vi "DT_GetDependencyFiles.vi"(7 "Framwork Type":T1) -> (1 "rel. Filepaths .js":path[](array[path]), 2 "rel. Filepaths .css":path[](array[path]))   [LabVIEW 2014]
uses:
  controls/StylingFrameworks_Enum.ctl
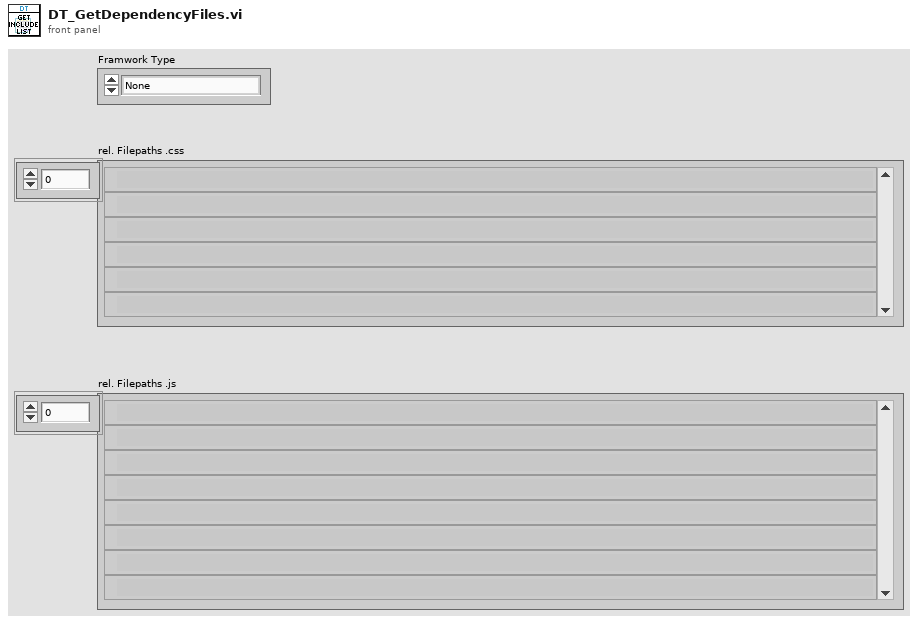
[diagram p1: front panel]
types:
  T1 = typedef "StylingFrameworks_Enum.ctl" = enum16{"None", "Bootstrap4", "Semantic-UI", "Custom"}
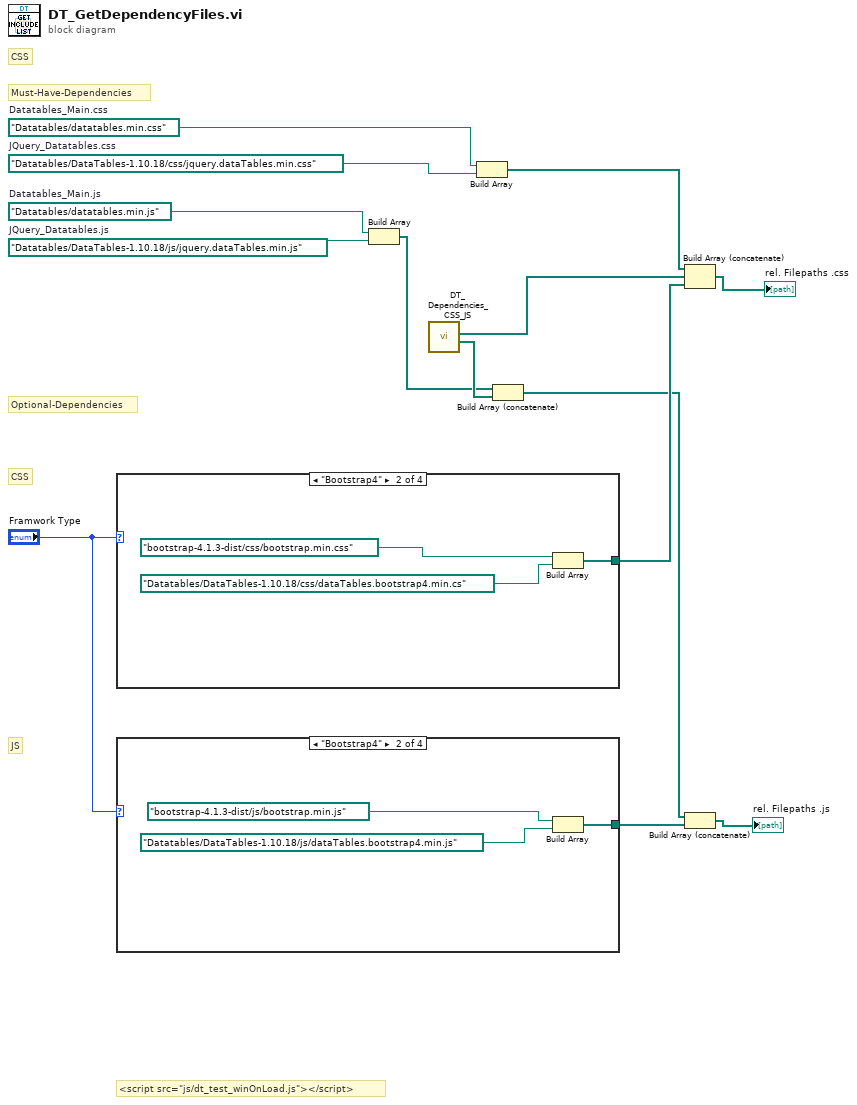
[diagram p0: block diagram]
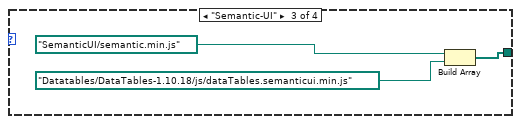
[diagram p3: hidden frame]
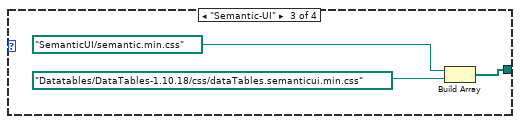
[diagram p6: hidden frame]
diagram:
  w6 = path "Datatables/DataTables-1.10.18/js/jquery.dataTables.min.js"  # JQuery_Datatables.js
  w7 = path "Datatables/datatables.min.js"  # Datatables_Main.js
  w10 = path "Datatables/DataTables-1.10.18/css/jquery.dataTables.min.css"  # JQuery_Datatables.css
  w12 = path "Datatables/datatables.min.css"  # Datatables_Main.css
  # "CSS"
  # "JS"
  # "CSS"
  # "<script src=\"js/dt_test_winOnLoad.js\"></script>"
  # "Optional-Dependencies"
  # "Must-Have-Dependencies"
  n1 = case shown="\"Bootstrap4\"" "Framwork Type" {
    tunnel: [_ w15 w18 _] -> w9
    frame "None", Default {
    }
    frame "Bootstrap4" {
      n2 = Build Array(path "bootstrap-4.1.3-dist/css/bootstrap.min.css", path "Datatables/DataTables-1.10.18/css/dataTables.bootstrap4.min.cs") -> (w15:path[])
    }
    frame "Semantic-UI" {
      n3 = Build Array(path "SemanticUI/semantic.min.css", path "Datatables/DataTables-1.10.18/css/dataTables.semanticui.min.css") -> (w18:path[])
    }
    frame "Custom" {
    }
  }
  n4 = case shown="\"Bootstrap4\"" "Framwork Type" {
    tunnel: [_ w21 w24 _] -> w13
    frame "None", Default {
    }
    frame "Bootstrap4" {
      n5 = Build Array(path "bootstrap-4.1.3-dist/js/bootstrap.min.js", path "Datatables/DataTables-1.10.18/js/dataTables.bootstrap4.min.js") -> (w21:path[])
    }
    frame "Semantic-UI" {
      n6 = Build Array(path "SemanticUI/semantic.min.js", path "Datatables/DataTables-1.10.18/js/dataTables.semanticui.min.js") -> (w24:path[])
    }
    frame "Custom" {
    }
  }
  n7 = Build Array(w7, w6) -> (w1:path[])
  n8 = call "DT_Dependencies_CSS_JS.vi"() -> ("DT_Extensions_JS_Files"=w4:path[], "DT_Extensions_CSS_Files"=w8:path[])  [unwired: 10 in]
  n9 = Build Array(w12, w10) -> (w11:path[])
  n10 = Build Array (concatenate)(w1, w4) -> (w5:path[])
  n11 = Build Array (concatenate)(w11, w8, w9) -> (→"rel. Filepaths .css":path[])
  n12 = Build Array (concatenate)(w5, w13) -> (→"rel. Filepaths .js":path[])
